vi "oax_Select Listbox.vi"(8 "error in":errorcluster, 10 "Item Names":string[](array[string])) -> (0 "error out":errorcluster, 2 "orders to extract out":dbl[](array[numeric]), 3 "File Path (.wav)":path=path "C:/Program Files/National Instruments/LabVIEW 8.2/examples/Order Analysis/Demo VI/Example Data/DownAcc.wav", 5 "OK?":bool)   [LabVIEW 2017]
panel:
  in  "Add orders listbox":i32[](listbox) caption="Select One Order"
  in  "Save Path (.wav)":path
  in  "Cancel":bool
  in  "OK":bool
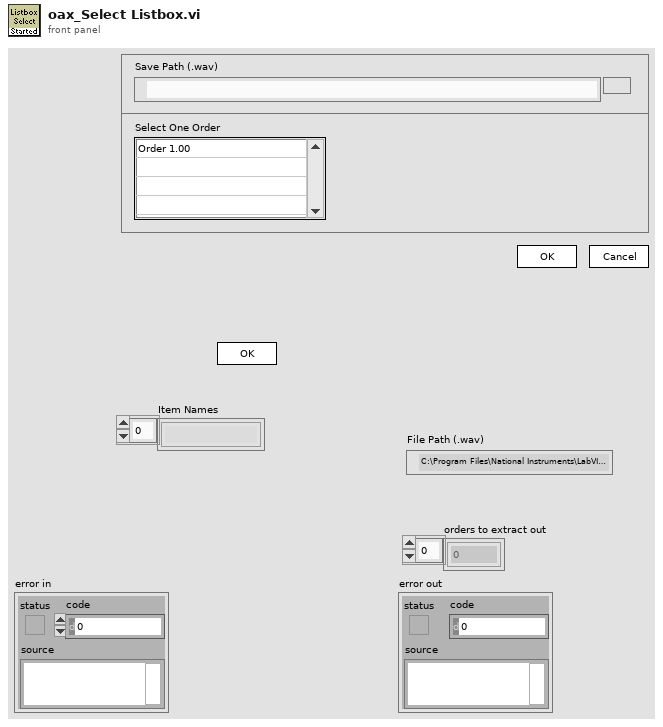
[diagram p1: front panel]
types:
  T1 = enum16{"Read", "Add", "Delete", "Clear", "GetSelected"}
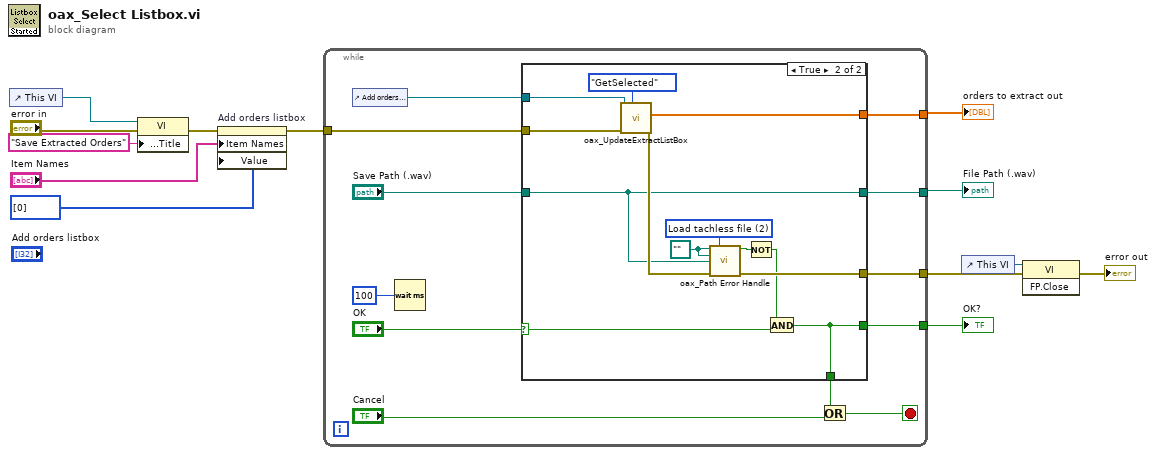
[diagram p0: block diagram]
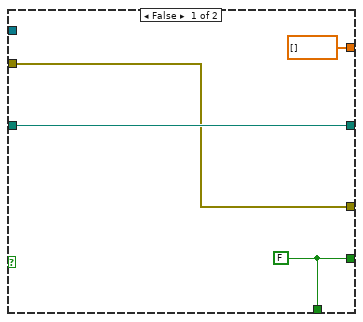
[diagram p2: hidden frame]
diagram:
  n1 = control-ref of="This VI"() -> (w5:refnum<vi>)
  n2 = property class="VI"(reference=w5, error in="error in", "Front Panel.Title"="Save Extracted Orders" ("Front Panel Window:Title")) -> (error out=w4:errorcluster)  [unwired: 1 out]
  n3 = property on="Add orders listbox" class="LstBox (strict)"(error in=w4, "Item Names"="Item Names", "Value"=i32[] [0] ("Add orders listbox")) -> (error out=w9:errorcluster)  [unwired: 1 in, 1 out]
  n4 = while {
    tunnel: [w23] -> w13
    tunnel: [w22] -> w12
    tunnel: [w21] -> w11
    tunnel: [w20] -> w10
    tunnel: w9 -> [w14]
    stop <- w17 stop-if-true
    n5 = control-ref of="Add orders listbox"() -> (w15:refnum<vi>)
    n6 = Wait (ms)(milliseconds to wait=u32 100) -> ()  [unwired: 1 out]
    n7 = case shown="True" "OK" {
      selector: "OK" -> [_ w38]
      tunnel: w14 -> [w27 w42]
      tunnel: "Save Path (.wav)" -> [w28 w34]
      tunnel: [w28 w34] -> w23
      tunnel: [dbl[] [] ("orders to extract out") w39] -> w22
      tunnel: [w26 w36] -> w21
      tunnel: [w27 w37] -> w20
      tunnel: [w26 w36] -> w16
      tunnel: w15 -> [_ w35]
      frame False {
        w26 = FALSE
      }
      frame True {
        w33 = path "" ("File Path (.dat)")
        w41 = u16 2 items=["Load .wav file", "Load .dat file", "Load tachless file"] ("Ring")
        n8 = call <vilib>:"oax_UpdateExtractListBox.vi"("operation"=T1."GetSelected", "error in (no error)"=w42, "ref in"=w35) -> ("error out"=w40:errorcluster, "orders to extract out"=w39:dbl[])  [unwired: 6 in, 1 out]
        n9 = call <vilib>:"oax_Path Error Handle.vi"("File Path (.dat)"=w33, "Ring"=w41, "Tacho File Path (.wav)"=w33, "Vibration File Path (.wav)"=w34, "error In"=w40) -> ("Error"=w32:bool, "error Out"=w37:errorcluster)  [unwired: 9 in]
        n10 = Not(x=w32) -> (.not. x?=w31:bool)
        n11 = And(x=w31, y=w38) -> (x .and. y?=w36:bool)
      }
    }
    n12 = Or(x=w16, y="Cancel") -> (x .or. y?=w17:bool)
  }
  "File Path (.wav)" <- w13
  "OK?" <- w11
  "orders to extract out" <- w12
  n13 = control-ref of="This VI"() -> (w7:refnum<vi>)
  n14 = invoke class="VI" method="FP.Close"(reference=w7, error in=w10) -> (error out=→"error out":errorcluster)  [unwired: 1 in, 2 out]
